vi "LvMPDC_SUB_ReadWriteConfigIni.vi"(6 "Read/Write(T)":bool, 8 "error in (no error)":errorcluster caption="エラー入力（エラーなし）", 9 "Config":T1, 11 "ConfigIni filepath":path=path "Config.ini") -> (0 "error out":errorcluster caption="エラー出力", 1 "Config out":T1)   [LabVIEW 2012]
uses:
  LvMPDC_Typdef_Setting.ctl
  <vilib>/Utility/config.llb/Write Key (String).vi
  <vilib>/Utility/config.llb/Write Key (I32).vi
  <vilib>/Utility/config.llb/Read Key (String).vi
  <vilib>/Utility/config.llb/Read Key (I32).vi
  <vilib>/Utility/config.llb/NI_LVConfig.lvlib
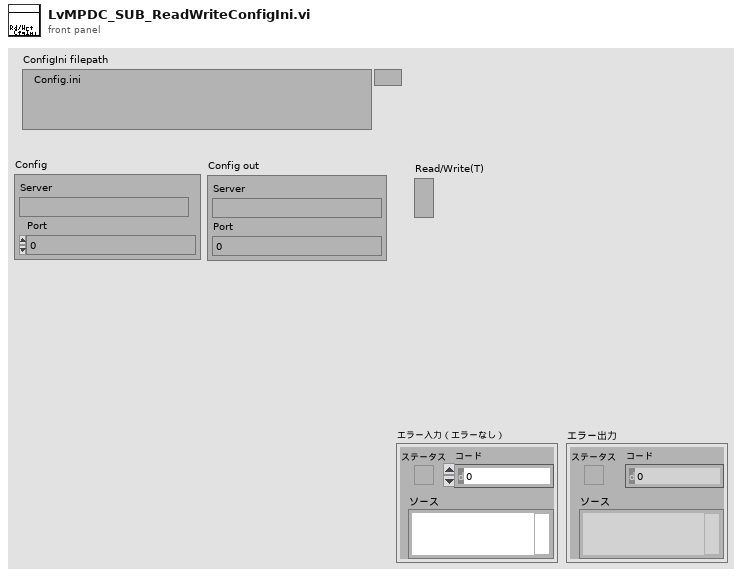
[diagram p1: front panel]
types:
  T1 = typedef "LvMPDC_Typdef_Setting.ctl" = cluster{"Server":string, "Port":u16}
  T2 = typedef "NI_LVConfig.lvlib/Config Data RefNum.ctl" = refnum<k1>
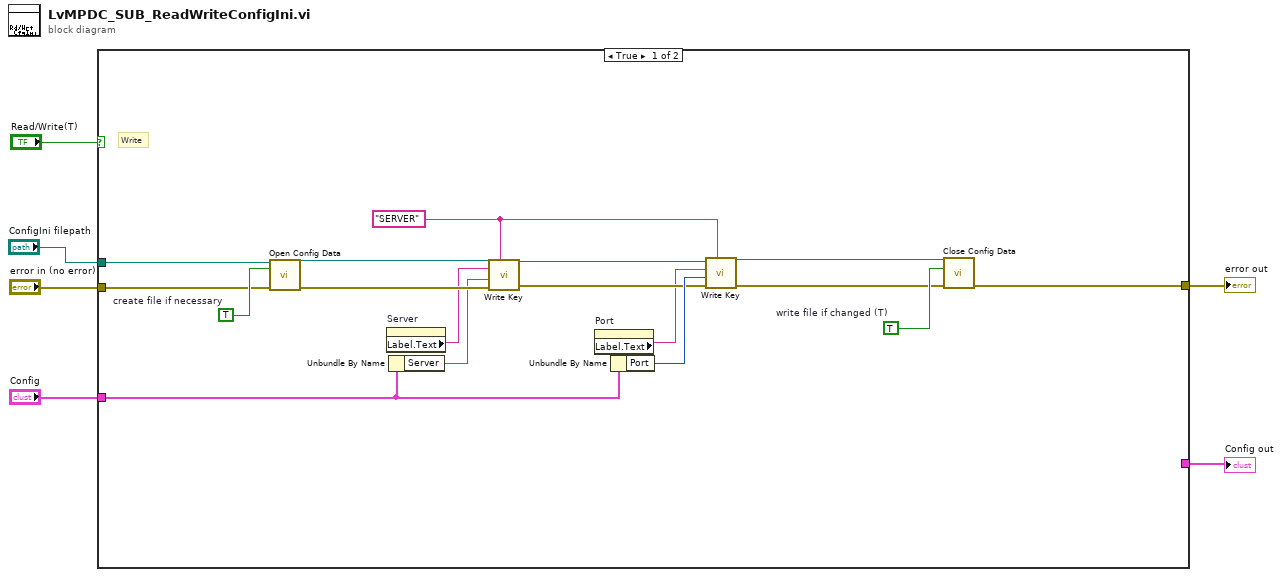
[diagram p0: block diagram]
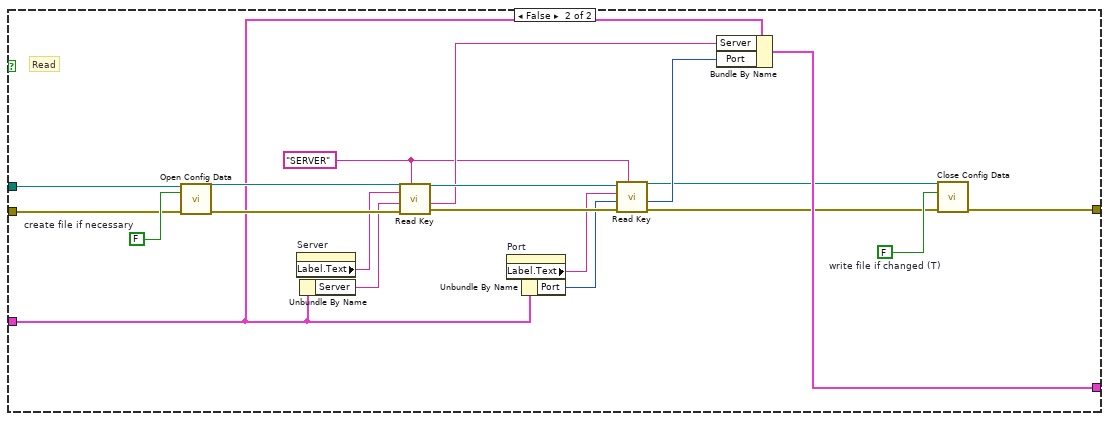
[diagram p2: hidden frame]
diagram:
  n1 = case shown="TRUE" "Read/Write(T)" {
    tunnel: "error in (no error)" -> [w22 w42]
    tunnel: [w20 w40] -> w5
    tunnel: "ConfigIni filepath" -> [w21 w41]
    tunnel: "Config" -> [w11 w29]
    tunnel: [_ w28] -> w1
    frame True {
      w12 = "SERVER"
      w19 = TRUE  # write file if changed (T)
      w23 = TRUE  # create file if necessary
      # "Write"
      n2 = call <vilib>:"Open Config Data.vi"("error in (no error)"=w22, "create file if necessary (T)"=w23, "configuration file path"=w21) -> ("error out"=w17:errorcluster, "refnum"=w18:T2)  [unwired: 6 in, 1 out]
      n3 = property on="Server" class="Str"() -> ("Label.Text"=w8:string)  [unwired: 2 in, 2 out]
      n4 = Unbundle By Name(w11) -> ("Server"=w16:string)
      n5 = call-poly <vilib>:"Write Key.vi"("section"=w12, "error in (no error)"=w17, "value"=w16, "key"=w8, "refnum"=w18) -> ("error out"=w14:errorcluster, "refnum out"=w13:T2)  [unwired: 4 in, 1 out]
      n6 = property on="Port" class="DigNum （指定）"() -> ("Label.Text"=w7:string)  [unwired: 2 in, 2 out]
      n7 = Unbundle By Name(w11) -> ("Port"=w15:u16)
      n8 = call-poly <vilib>:"Write Key.vi"("section"=w12, "error in (no error)"=w14, "value"=w15, "key"=w7, "refnum"=w13) -> ("error out"=w9:errorcluster, "refnum out"=w10:T2)  [unwired: 4 in, 1 out]
      n9 = call <vilib>:"Close Config Data.vi"("error in (no error)"=w9, "write file if changed (T)"=w19, "refnum"=w10) -> ("error out"=w20:errorcluster)  [unwired: 7 in, 1 out]
    }
    frame False {
      w30 = "SERVER"
      w39 = FALSE  # write file if changed (T)
      w43 = FALSE  # create file if necessary
      # "Read"
      n10 = call <vilib>:"Open Config Data.vi"("error in (no error)"=w42, "create file if necessary (T)"=w43, "configuration file path"=w41) -> ("error out"=w37:errorcluster, "refnum"=w38:T2)  [unwired: 6 in, 1 out]
      n11 = property on="Server" class="Str"() -> ("Label.Text"=w25:string)  [unwired: 2 in, 2 out]
      n12 = Unbundle By Name(w29) -> ("Server"=w34:string)
      n13 = call-poly <vilib>:"Read Key.vi"("section"=w30, "error in (no error)"=w37, "default value"=w34, "key"=w25, "refnum"=w38) -> ("error out"=w36:errorcluster, "value"=w32:string, "refnum out"=w35:T2)  [unwired: 3 in, 1 out]
      n14 = property on="Port" class="DigNum （指定）"() -> ("Label.Text"=w24:string)  [unwired: 2 in, 2 out]
      n15 = Unbundle By Name(w29) -> ("Port"=w33:u16)
      n16 = call-poly <vilib>:"Read Key.vi"("section"=w30, "error in (no error)"=w36, "default value"=w33, "key"=w24, "refnum"=w35) -> ("error out"=w26:errorcluster, "value"=w31:i32, "refnum out"=w27:T2)  [unwired: 3 in, 1 out]
      n17 = Bundle By Name(cluster=w29, "Server"=w32, "Port"=w31) -> (w28:T1)
      n18 = call <vilib>:"Close Config Data.vi"("error in (no error)"=w26, "write file if changed (T)"=w39, "refnum"=w27) -> ("error out"=w40:errorcluster)  [unwired: 7 in, 1 out]
    }
  }
  "error out" <- w5
  "Config out" <- w1
